vi "Test for 7841.vi"() -> ()   [LabVIEW 2018]
uses:
  <vilib>/Platform/TimedLoop/XDataNode/timing_clust.ctl
  <vilib>/Platform/TimedLoop/XDataNode/nitl_modes.ctl
  <vilib>/Platform/TimedLoop/XDataNode/wakeup.ctl
  <vilib>/rvi/Emulation/niFpgaGetClockAttributes.vi
  <vilib>/rvi/Emulation/niFpgaSctlEmulationGetInTimedLoop.vi
  <vilib>/rvi/Emulation/niFpgaEmulationReportErrorSimple.vi
  <vilib>/rvi/Emulation/niFpgaProcessEmulError.vi
  <vilib>/rvi/eio/common/nirviEmuTemplateMethod_errors.vi
  <vilib>/rvi/Emulation/niFpgaCriticalErrorInLSC.vi
  <vilib>/eio/EIONode/EIONode.xnode
  <vilib>/Platform/TimedLoop/XDataNode/XDataNode.xnode
  <vilib>/Platform/TimedLoop/XDataNode/XDNodeRunTimeDep.lvlib
panel:
  in  "Connector0/DIO15":bool
  in  "Connector0/DIO14":bool
  in  "Connector0/DIO13":bool
  in  "Connector0/DIO12":bool
  in  "Connector0/DIO11":bool
  in  "Connector0/DIO10":bool
  in  "Connector0/DIO9":bool
  in  "Connector0/DIO8":bool
  in  "Connector0/DIO7":bool
  in  "Connector0/DIO6":bool
  in  "Connector0/DIO5":bool
  in  "Connector0/DIO4":bool
  in  "Connector0/DIO3":bool
  in  "Connector0/DIO2":bool
  in  "Connector0/DIO1":bool
  in  "Connector0/DIO0":bool
  in  "Connector2/DIO0":bool
  in  "Connector2/DIO1":bool
  in  "Connector2/DIO2":bool
  in  "Connector2/DIO3":bool
  in  "Connector2/DIO4":bool
  in  "Connector2/DIO5":bool
  in  "Connector2/DIO6":bool
  in  "Connector2/DIO7":bool
  in  "Connector2/DIO8":bool
  in  "Connector2/DIO9":bool
  in  "Connector2/DIO10":bool
  in  "Connector2/DIO11":bool
  in  "Connector2/DIO12":bool
  in  "Connector2/DIO13":bool
  in  "Connector2/DIO14":bool
  in  "Connector2/DIO15":bool
  in  "Connector2/DIO16":bool
  in  "Connector2/DIO17":bool
  in  "Connector2/DIO18":bool
  in  "Connector2/DIO19":bool
  in  "Connector2/DIO20":bool
  in  "Connector2/DIO21":bool
  in  "Connector2/DIO22":bool
  in  "Connector2/DIO23":bool
  in  "Connector2/DIO24":bool
  in  "Connector2/DIO25":bool
  in  "Connector2/DIO26":bool
  in  "Connector2/DIO27":bool
  in  "Connector2/DIO28":bool
  in  "Connector2/DIO29":bool
  in  "Connector2/DIO30":bool
  in  "Connector2/DIO31":bool
  in  "Connector2/DIO32":bool
  in  "Connector2/DIO33":bool
  in  "Connector2/DIO34":bool
  in  "Connector2/DIO35":bool
  in  "Connector2/DIO36":bool
  in  "Connector2/DIO37":bool
  in  "Connector2/DIO38":bool
  in  "Connector2/DIO39":bool
  in  "Connector1/DIO39":bool
  in  "Connector1/DIO38":bool
  in  "Connector1/DIO37":bool
  in  "Connector1/DIO36":bool
  in  "Connector1/DIO35":bool
  in  "Connector1/DIO34":bool
  in  "Connector1/DIO33":bool
  in  "Connector1/DIO32":bool
  in  "Connector1/DIO31":bool
  in  "Connector1/DIO30":bool
  in  "Connector1/DIO29":bool
  in  "Connector1/DIO28":bool
  in  "Connector1/DIO27":bool
  in  "Connector1/DIO26":bool
  in  "Connector1/DIO25":bool
  in  "Connector1/DIO24":bool
  in  "Connector1/DIO23":bool
  in  "Connector1/DIO22":bool
  in  "Connector1/DIO21":bool
  in  "Connector1/DIO20":bool
  in  "Connector1/DIO19":bool
  in  "Connector1/DIO18":bool
  in  "Connector1/DIO17":bool
  in  "Connector1/DIO16":bool
  in  "Connector1/DIO15":bool
  in  "Connector1/DIO14":bool
  in  "Connector1/DIO13":bool
  in  "Connector1/DIO12":bool
  in  "Connector1/DIO11":bool
  in  "Connector1/DIO10":bool
  in  "Connector1/DIO9":bool
  in  "Connector1/DIO8":bool
  in  "Connector1/DIO7":bool
  in  "Connector1/DIO6":bool
  in  "Connector1/DIO5":bool
  in  "Connector1/DIO4":bool
  in  "Connector1/DIO3":bool
  in  "Connector1/DIO2":bool
  in  "Connector1/DIO1":bool
  in  "Connector1/DIO0":bool
  out "Connector0/AI7":i16
  out "Connector0/AI6":i16
  out "Connector0/AI5":i16
  out "Connector0/AI4":i16
  out "Connector0/AI3":i16
  out "Connector0/AI2":i16
  out "Connector0/AI1":i16
  out "Connector0/AI0":i16
  in  "Connector0/AO7":i16
  in  "Connector0/AO6":i16
  in  "Connector0/AO5":i16
  in  "Connector0/AO4":i16
  in  "Connector0/AO3":i16
  in  "Connector0/AO2":i16
  in  "Connector0/AO1":i16
  in  "Connector0/AO0":i16
  in  "Стоп":bool
  in  "Constant(F) / Frequency(T)":bool
  in  "Devider Frequency 160/(x*2), x>0":u8=1 min=1
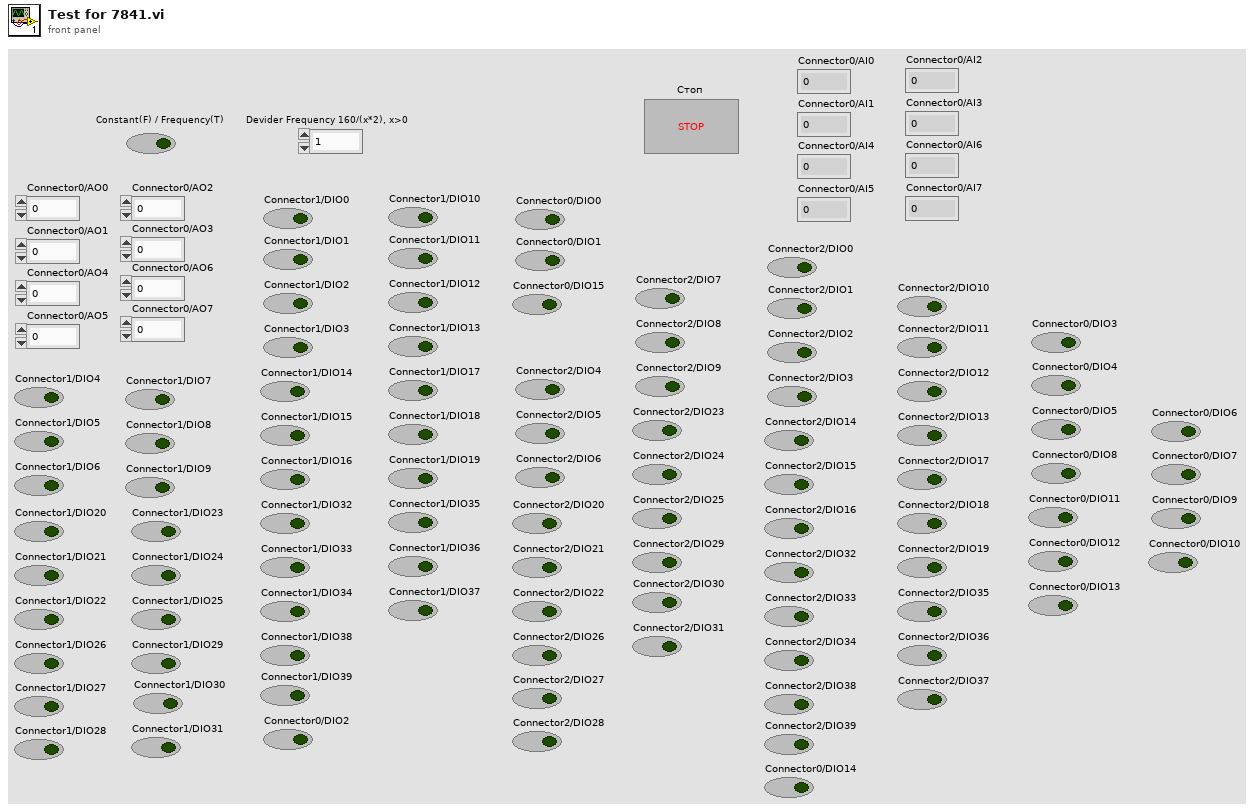
[diagram p1: front panel]
types:
  T1 = typedef "XDNodeRunTimeDep.lvlib/timing_clust.ctl" = cluster{"Expected End [f-1]":u64, "Actual End [f-1]":u64, "Finished Late? [f-1]":bool, "Expected End [i-1]":u64, "Actual End [i-1]":u64, "Finished Late? [i-1]":bool, "Expected Start [i]":u64, "Actual Start [i]":u64, "Expected Start [f]":u64, "Actual Start [f]":u64, "Source Name":string, "Structure Name":string, "Period":i64, "Deadline":i64, "Offset":i64, "Start":i64, "Priority":i32, "Timeout":i32, "Mode":T2, "Wakeup Reason":T3, "Error":errorcluster, "Source Type":string, "Secondary Source Type":string, "Global End Time":u64, "Global Start Time":u64, "Frame Duration":u64, "Iteration Duration":u64, "Assigned CPU":i32, "I/O Scan Engine Mode":u32}
  T2 = typedef "XDNodeRunTimeDep.lvlib/nitl_modes.ctl" = enum32{"No Change", "Process missed periods, maintain original phase", "Discard missed periods, maintain original phase", "Process missed periods, ignore original phase", "Discard missed periods, ignore original phase"}
  T3 = typedef "XDNodeRunTimeDep.lvlib/wakeup.ctl" = enum32{"Normal", "Aborted", "Asynchronous wakeup", "Timing source error", "Timed loop error", "Timeout"}
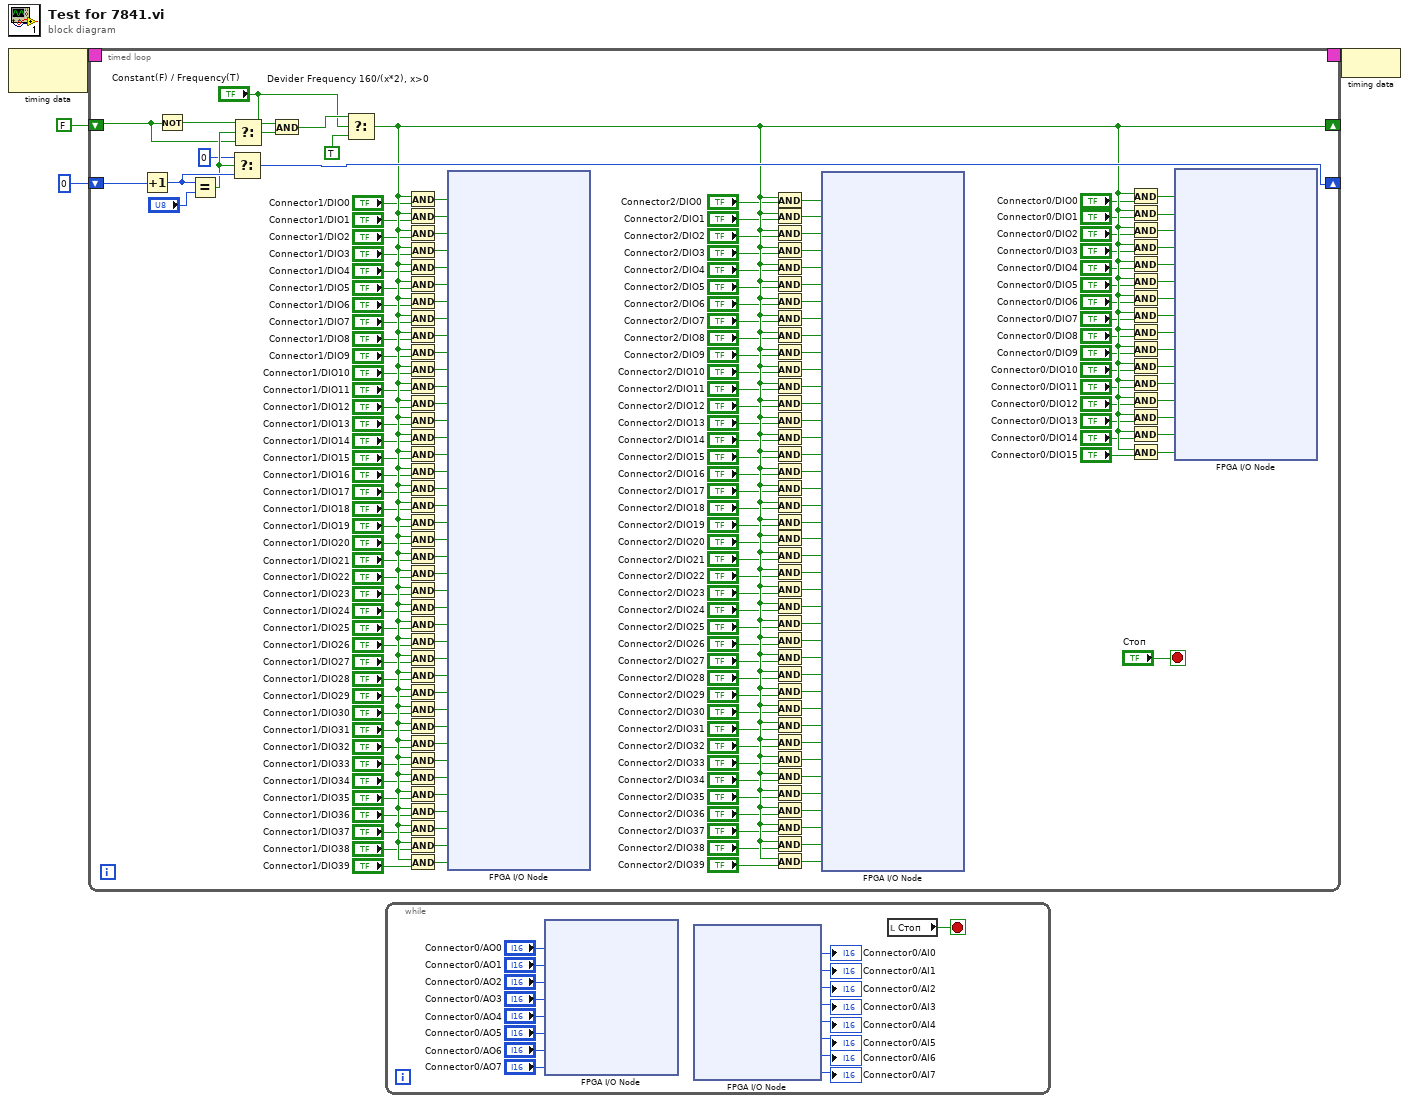
[diagram p0: block diagram]
diagram:
  n1 = node-c288() -> (w4:T1)  [unwired: 1 in]
  n2 = timed-loop {
    timing: w4 -> [_]
    timing-out: [_] -> w3
    shift-right: [w197] -> _
    shift-left: FALSE -> [w203]
    shift-right: [w201] -> _
    shift-left: u8 0 -> [w202]
    stop <- "Стоп" stop-if-true
    n3 = Increment(x=w202) -> (x+1=w207:u8)
    n4 = Not(x=w203) -> (.not. x?=w209:bool)
    n5 = Equal?(x=w207, y="Devider Frequency 160/(x*2), x>0") -> (x = y?=w206:bool)
    n6 = Select(t=u8 0, s=w206, f=w207) -> (s? t:f=w201:u8)
    n7 = Select(t=w209, s=w206, f=w203) -> (s? t:f=w204:bool)
    n8 = And(x="Constant(F) / Frequency(T)", y=w204) -> (x .and. y?=w200:bool)
    n9 = Select(t=w200, s="Constant(F) / Frequency(T)", f=TRUE ("t")) -> (s? t:f=w197:bool)
    n10 = And(x=w197, y="Connector1/DIO0") -> (x .and. y?=w194:bool)
    n11 = And(x=w197, y="Connector1/DIO1") -> (x .and. y?=w192:bool)
    n12 = And(x=w197, y="Connector1/DIO2") -> (x .and. y?=w191:bool)
    n13 = And(x=w197, y="Connector1/DIO3") -> (x .and. y?=w189:bool)
    n14 = And(x=w197, y="Connector1/DIO4") -> (x .and. y?=w187:bool)
    n15 = And(x=w197, y="Connector1/DIO5") -> (x .and. y?=w185:bool)
    n16 = And(x=w197, y="Connector1/DIO6") -> (x .and. y?=w183:bool)
    n17 = And(x=w197, y="Connector1/DIO7") -> (x .and. y?=w181:bool)
    n18 = And(x=w197, y="Connector1/DIO8") -> (x .and. y?=w179:bool)
    n19 = And(x=w197, y="Connector1/DIO9") -> (x .and. y?=w177:bool)
    n20 = And(x=w197, y="Connector1/DIO10") -> (x .and. y?=w175:bool)
    n21 = And(x=w197, y="Connector1/DIO11") -> (x .and. y?=w173:bool)
    n22 = And(x=w197, y="Connector1/DIO12") -> (x .and. y?=w171:bool)
    n23 = And(x=w197, y="Connector1/DIO13") -> (x .and. y?=w169:bool)
    n24 = And(x=w197, y="Connector1/DIO14") -> (x .and. y?=w167:bool)
    n25 = And(x=w197, y="Connector1/DIO15") -> (x .and. y?=w165:bool)
    n26 = And(x=w197, y="Connector1/DIO16") -> (x .and. y?=w163:bool)
    n27 = And(x=w197, y="Connector1/DIO17") -> (x .and. y?=w161:bool)
    n28 = And(x=w197, y="Connector1/DIO18") -> (x .and. y?=w159:bool)
    n29 = And(x=w197, y="Connector1/DIO19") -> (x .and. y?=w157:bool)
    n30 = And(x=w197, y="Connector1/DIO20") -> (x .and. y?=w155:bool)
    n31 = And(x=w197, y="Connector1/DIO21") -> (x .and. y?=w153:bool)
    n32 = And(x=w197, y="Connector1/DIO22") -> (x .and. y?=w151:bool)
    n33 = And(x=w197, y="Connector1/DIO23") -> (x .and. y?=w149:bool)
    n34 = And(x=w197, y="Connector1/DIO24") -> (x .and. y?=w147:bool)
    n35 = And(x=w197, y="Connector1/DIO25") -> (x .and. y?=w145:bool)
    n36 = And(x=w197, y="Connector1/DIO26") -> (x .and. y?=w143:bool)
    n37 = And(x=w197, y="Connector1/DIO27") -> (x .and. y?=w141:bool)
    n38 = And(x=w197, y="Connector1/DIO28") -> (x .and. y?=w139:bool)
    n39 = And(x=w197, y="Connector1/DIO29") -> (x .and. y?=w137:bool)
    n40 = And(x=w197, y="Connector1/DIO30") -> (x .and. y?=w135:bool)
    n41 = And(x=w197, y="Connector1/DIO31") -> (x .and. y?=w133:bool)
    n42 = And(x=w197, y="Connector1/DIO32") -> (x .and. y?=w131:bool)
    n43 = And(x=w197, y="Connector1/DIO33") -> (x .and. y?=w129:bool)
    n44 = And(x=w197, y="Connector1/DIO34") -> (x .and. y?=w127:bool)
    n45 = And(x=w197, y="Connector1/DIO35") -> (x .and. y?=w125:bool)
    n46 = And(x=w197, y="Connector1/DIO36") -> (x .and. y?=w123:bool)
    n47 = And(x=w197, y="Connector1/DIO37") -> (x .and. y?=w121:bool)
    n48 = And(x=w197, y="Connector1/DIO38") -> (x .and. y?=w119:bool)
    n49 = And(x=w197, y="Connector1/DIO39") -> (x .and. y?=w117:bool)
    n50 = xnode "FPGA I/O Node"("Connector1/DIO0"=w194, "Connector1/DIO1"=w192, "Connector1/DIO2"=w191, "Connector1/DIO3"=w189, "Connector1/DIO4"=w187, "Connector1/DIO5"=w185, "Connector1/DIO6"=w183, "Connector1/DIO7"=w181, "Connector1/DIO8"=w179, "Connector1/DIO9"=w177, "Connector1/DIO10"=w175, "Connector1/DIO11"=w173, "Connector1/DIO12"=w171, "Connector1/DIO13"=w169, "Connector1/DIO14"=w167, "Connector1/DIO15"=w165, "Connector1/DIO16"=w163, "Connector1/DIO17"=w161, "Connector1/DIO18"=w159, "Connector1/DIO19"=w157, "Connector1/DIO20"=w155, "Connector1/DIO21"=w153, "Connector1/DIO22"=w151, "Connector1/DIO23"=w149, "Connector1/DIO24"=w147, "Connector1/DIO25"=w145, "Connector1/DIO26"=w143, "Connector1/DIO27"=w141, "Connector1/DIO28"=w139, "Connector1/DIO29"=w137, "Connector1/DIO30"=w135, "Connector1/DIO31"=w133, "Connector1/DIO32"=w131, "Connector1/DIO33"=w129, "Connector1/DIO34"=w127, "Connector1/DIO35"=w125, "Connector1/DIO36"=w123, "Connector1/DIO37"=w121, "Connector1/DIO38"=w119, "Connector1/DIO39"=w117) -> ()  [unwired: 40 in, 40 out]
    n51 = And(x=w197, y="Connector2/DIO0") -> (x .and. y?=w116:bool)
    n52 = And(x=w197, y="Connector2/DIO1") -> (x .and. y?=w115:bool)
    n53 = And(x=w197, y="Connector2/DIO2") -> (x .and. y?=w114:bool)
    n54 = And(x=w197, y="Connector2/DIO3") -> (x .and. y?=w113:bool)
    n55 = And(x=w197, y="Connector2/DIO4") -> (x .and. y?=w112:bool)
    n56 = And(x=w197, y="Connector2/DIO5") -> (x .and. y?=w111:bool)
    n57 = And(x=w197, y="Connector2/DIO6") -> (x .and. y?=w110:bool)
    n58 = And(x=w197, y="Connector2/DIO7") -> (x .and. y?=w109:bool)
    n59 = And(x=w197, y="Connector2/DIO8") -> (x .and. y?=w108:bool)
    n60 = And(x=w197, y="Connector2/DIO9") -> (x .and. y?=w107:bool)
    n61 = And(x=w197, y="Connector2/DIO10") -> (x .and. y?=w106:bool)
    n62 = And(x=w197, y="Connector2/DIO11") -> (x .and. y?=w105:bool)
    n63 = And(x=w197, y="Connector2/DIO12") -> (x .and. y?=w104:bool)
    n64 = And(x=w197, y="Connector2/DIO13") -> (x .and. y?=w103:bool)
    n65 = And(x=w197, y="Connector2/DIO14") -> (x .and. y?=w102:bool)
    n66 = And(x=w197, y="Connector2/DIO15") -> (x .and. y?=w101:bool)
    n67 = And(x=w197, y="Connector2/DIO16") -> (x .and. y?=w100:bool)
    n68 = And(x=w197, y="Connector2/DIO17") -> (x .and. y?=w99:bool)
    n69 = And(x=w197, y="Connector2/DIO18") -> (x .and. y?=w98:bool)
    n70 = And(x=w197, y="Connector2/DIO19") -> (x .and. y?=w97:bool)
    n71 = And(x=w197, y="Connector2/DIO20") -> (x .and. y?=w96:bool)
    n72 = And(x=w197, y="Connector2/DIO21") -> (x .and. y?=w95:bool)
    n73 = And(x=w197, y="Connector2/DIO22") -> (x .and. y?=w94:bool)
    n74 = And(x=w197, y="Connector2/DIO23") -> (x .and. y?=w93:bool)
    n75 = And(x=w197, y="Connector2/DIO24") -> (x .and. y?=w92:bool)
    n76 = And(x=w197, y="Connector2/DIO25") -> (x .and. y?=w91:bool)
    n77 = And(x=w197, y="Connector2/DIO26") -> (x .and. y?=w90:bool)
    n78 = And(x=w197, y="Connector2/DIO27") -> (x .and. y?=w89:bool)
    n79 = And(x=w197, y="Connector2/DIO28") -> (x .and. y?=w88:bool)
    n80 = And(x=w197, y="Connector2/DIO29") -> (x .and. y?=w87:bool)
    n81 = And(x=w197, y="Connector2/DIO30") -> (x .and. y?=w86:bool)
    n82 = And(x=w197, y="Connector2/DIO31") -> (x .and. y?=w85:bool)
    n83 = And(x=w197, y="Connector2/DIO32") -> (x .and. y?=w84:bool)
    n84 = And(x=w197, y="Connector2/DIO33") -> (x .and. y?=w83:bool)
    n85 = And(x=w197, y="Connector2/DIO34") -> (x .and. y?=w82:bool)
    n86 = And(x=w197, y="Connector2/DIO35") -> (x .and. y?=w81:bool)
    n87 = And(x=w197, y="Connector2/DIO36") -> (x .and. y?=w80:bool)
    n88 = And(x=w197, y="Connector2/DIO37") -> (x .and. y?=w79:bool)
    n89 = And(x=w197, y="Connector2/DIO38") -> (x .and. y?=w78:bool)
    n90 = And(x=w197, y="Connector2/DIO39") -> (x .and. y?=w77:bool)
    n91 = xnode "FPGA I/O Node"("Connector2/DIO0"=w116, "Connector2/DIO1"=w115, "Connector2/DIO2"=w114, "Connector2/DIO3"=w113, "Connector2/DIO4"=w112, "Connector2/DIO5"=w111, "Connector2/DIO6"=w110, "Connector2/DIO7"=w109, "Connector2/DIO8"=w108, "Connector2/DIO9"=w107, "Connector2/DIO10"=w106, "Connector2/DIO11"=w105, "Connector2/DIO12"=w104, "Connector2/DIO13"=w103, "Connector2/DIO14"=w102, "Connector2/DIO15"=w101, "Connector2/DIO16"=w100, "Connector2/DIO17"=w99, "Connector2/DIO18"=w98, "Connector2/DIO19"=w97, "Connector2/DIO20"=w96, "Connector2/DIO21"=w95, "Connector2/DIO22"=w94, "Connector2/DIO23"=w93, "Connector2/DIO24"=w92, "Connector2/DIO25"=w91, "Connector2/DIO26"=w90, "Connector2/DIO27"=w89, "Connector2/DIO28"=w88, "Connector2/DIO29"=w87, "Connector2/DIO30"=w86, "Connector2/DIO31"=w85, "Connector2/DIO32"=w84, "Connector2/DIO33"=w83, "Connector2/DIO34"=w82, "Connector2/DIO35"=w81, "Connector2/DIO36"=w80, "Connector2/DIO37"=w79, "Connector2/DIO38"=w78, "Connector2/DIO39"=w77) -> ()  [unwired: 40 in, 40 out]
    n92 = And(x=w197, y="Connector0/DIO0") -> (x .and. y?=w76:bool)
    n93 = And(x=w197, y="Connector0/DIO1") -> (x .and. y?=w74:bool)
    n94 = And(x=w197, y="Connector0/DIO2") -> (x .and. y?=w73:bool)
    n95 = And(x=w197, y="Connector0/DIO3") -> (x .and. y?=w72:bool)
    n96 = And(x=w197, y="Connector0/DIO4") -> (x .and. y?=w71:bool)
    n97 = And(x=w197, y="Connector0/DIO5") -> (x .and. y?=w70:bool)
    n98 = And(x=w197, y="Connector0/DIO6") -> (x .and. y?=w69:bool)
    n99 = And(x=w197, y="Connector0/DIO7") -> (x .and. y?=w68:bool)
    n100 = And(x=w197, y="Connector0/DIO8") -> (x .and. y?=w67:bool)
    n101 = And(x=w197, y="Connector0/DIO9") -> (x .and. y?=w66:bool)
    n102 = And(x=w197, y="Connector0/DIO10") -> (x .and. y?=w65:bool)
    n103 = And(x=w197, y="Connector0/DIO11") -> (x .and. y?=w64:bool)
    n104 = And(x=w197, y="Connector0/DIO12") -> (x .and. y?=w63:bool)
    n105 = And(x=w197, y="Connector0/DIO13") -> (x .and. y?=w62:bool)
    n106 = And(x=w197, y="Connector0/DIO14") -> (x .and. y?=w61:bool)
    n107 = And(x=w197, y="Connector0/DIO15") -> (x .and. y?=w75:bool)
    n108 = xnode "FPGA I/O Node"("Connector0/DIO0"=w76, "Connector0/DIO1"=w74, "Connector0/DIO2"=w73, "Connector0/DIO3"=w72, "Connector0/DIO4"=w71, "Connector0/DIO5"=w70, "Connector0/DIO6"=w69, "Connector0/DIO7"=w68, "Connector0/DIO8"=w67, "Connector0/DIO9"=w66, "Connector0/DIO10"=w65, "Connector0/DIO11"=w64, "Connector0/DIO12"=w63, "Connector0/DIO13"=w62, "Connector0/DIO14"=w61, "Connector0/DIO15"=w75) -> ()  [unwired: 16 in, 16 out]
  }
  n109 = while {
    stop <- w229 stop-if-true
    n110 = xnode "FPGA I/O Node"("Connector0/AO0"="Connector0/AO0", "Connector0/AO1"="Connector0/AO1", "Connector0/AO2"="Connector0/AO2", "Connector0/AO3"="Connector0/AO3", "Connector0/AO4"="Connector0/AO4", "Connector0/AO5"="Connector0/AO5", "Connector0/AO6"="Connector0/AO6", "Connector0/AO7"="Connector0/AO7") -> ()  [unwired: 8 in, 8 out]
    n111 = xnode "FPGA I/O Node"() -> ("Connector0/AI0"=→"Connector0/AI0":i16, "Connector0/AI1"=→"Connector0/AI1":i16, "Connector0/AI2"=→"Connector0/AI2":i16, "Connector0/AI3"=→"Connector0/AI3":i16, "Connector0/AI4"=→"Connector0/AI4":i16, "Connector0/AI5"=→"Connector0/AI5":i16, "Connector0/AI6"=→"Connector0/AI6":i16, "Connector0/AI7"=→"Connector0/AI7":i16)  [unwired: 8 in, 8 out]
    n112 = local read "Стоп"() -> (w229:bool)
  }
  n113 = node-c288(w3) -> ()
